vi "Controller.vi"   [LabVIEW 2014, in "Controller Library.lvlib" / "Controller.lvclass"]
uses:
  Controller.lvclass
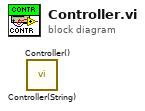
[diagram p0: block diagram]
diagram:
  n1 = call "Controller(String).vi"() -> ()  [unwired: 10 in, 2 out]
  n2 = call "Controller().vi"() -> ()  [unwired: 10 in, 2 out]
